vi "Dialog GraphSetting (Chart).vi"(11 "波形チャートref(in)":refnum<vi>) -> ()   [LabVIEW 2016]
uses:
  TypeDef/GraphSetting Appearance.ctl
  TypeDef/GraphSetting Plot.ctl
  SupportVIs/GraphSetting Scale.ctl
  TypeDef/GraphSetting DisplayFormatType.ctl
  TypeDef/GraphSetting All.ctl
  TypeDef/GraphSetting Command.ctl
  Library/Event/Write User Event (Array).vi
  <vilib>/Utility/xml.llb/Write to XML File(string).vi
  <vilib>/Utility/xml.llb/Read From XML File(string).vi
panel:
  in  "ファイル読込":bool
  in  "ファイル保存":bool
  in  "タブ制御器":enum32{"外観", "スケール", "プロット"}(tab)
  in  "外観":T1
  in  "Yスケール選択":u16(ring) items=["振幅"]
  in  "スケール(Y軸)":T2
  in  "スケール(X軸)":T2
  in  "Xスケール選択":u16(ring) items=["時間"]
  in  "プロット":T4 {"Yスケール" items=["振幅"]; "Xスケール" items=["時間"]; "プロット補間" max=5 step=1; "ポイントスタイル" max=16 step=1; "太さ" max=5 step=1; "ラインスタイル" max=4 step=1}
  in  "プロット選択":u16(ring) items=["正弦波", "プロット1"]
  in  "停止ボタン":bool
  # "欄外、パラメータ"
  # "スケールのスタイルとカラー"
  # "スケール係数"
  # "スケールのスタイルとカラー"
  # "スケールのスタイルとカラー"
  # "スケール係数"
  # "スケールのスタイルとカラー"
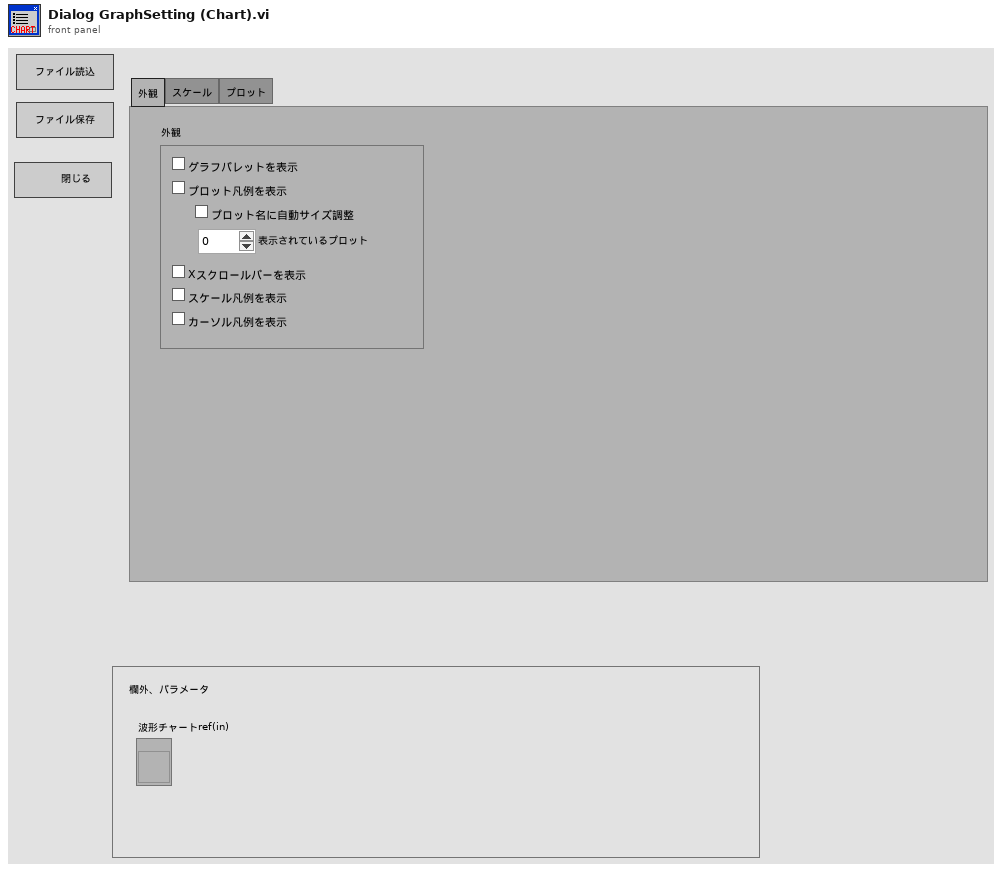
[diagram p1: front panel]
types:
  T1 = typedef "GraphSetting Appearance.ctl" = cluster{"グラフパレットを表示":bool, "プロット凡例を表示":bool, "プロット名に自動サイズ調整":bool, "表示されているプロット":u32, "Xスクロールバーを表示":bool, "スケール凡例を表示":bool, "カーソル凡例を表示":bool}
  T2 = typedef "GraphSetting Scale.ctl" = cluster{"名前":string, "スケールラベルを表示":bool, "スケールを表示":bool, "ログ":bool, "反転":bool, "自動スケール":bool, "最小":dbl, "最大":dbl, "オフセット":dbl, "乗数":dbl, "主目盛り":u32, "補助目盛り":u32, "マーカテキスト":u32, "主グリッド":u32, "補助グリッド":u32, "タイプ":T3, "小数点以下桁数":u8}
  T3 = typedef "GraphSetting DisplayFormatType.ctl" = enum8{"浮動小数点", "科学", "工学", "バイナリ", "８進数", "１６進数", "相対時間", "時間と日時", "SI"}
  T4 = typedef "GraphSetting Plot.ctl" = cluster{"名前":string, "表示":bool, "ラインスタイル":u8, "太さ":u8, "ポイントスタイル":u8, "プロット補間":u8, "ラインカラー":u32, "ポイント/塗りつぶし":u32, "Xスケール":u16, "Yスケール":u16}
  T5 = typedef "GraphSetting All.ctl" = cluster{"外観":T1, "スケールX[]":T2[], "スケールY[]":T2[], "プロット[]":T4[]}
  T6 = typedef "GraphSetting Command.ctl" = enum16{"Get(ref->ctl)", "Set(ctl->ref)"}
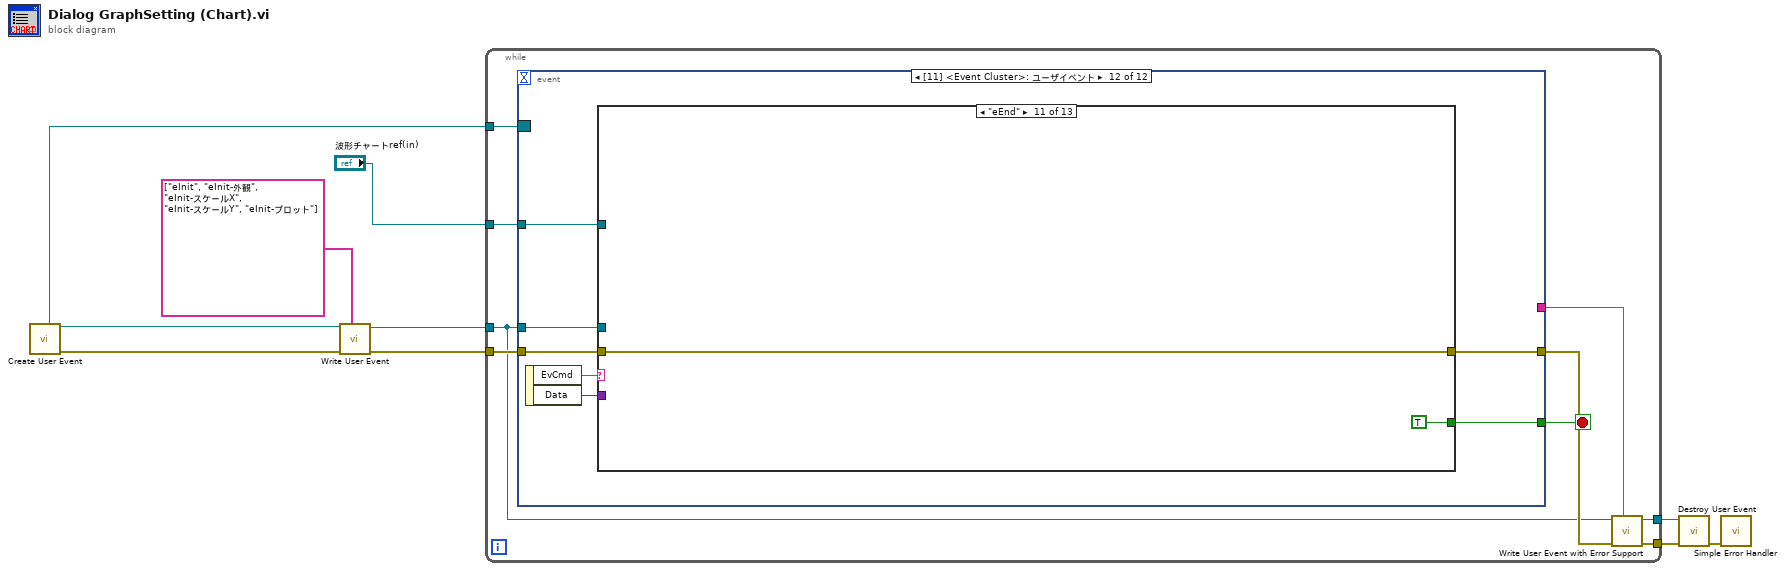
[diagram p0: block diagram]
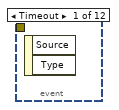
[diagram p2: hidden frame]
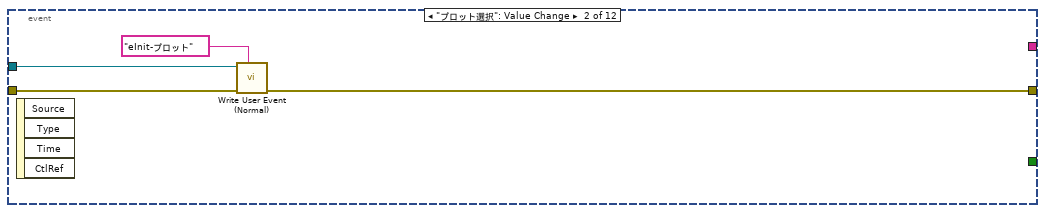
[diagram p3: hidden frame]
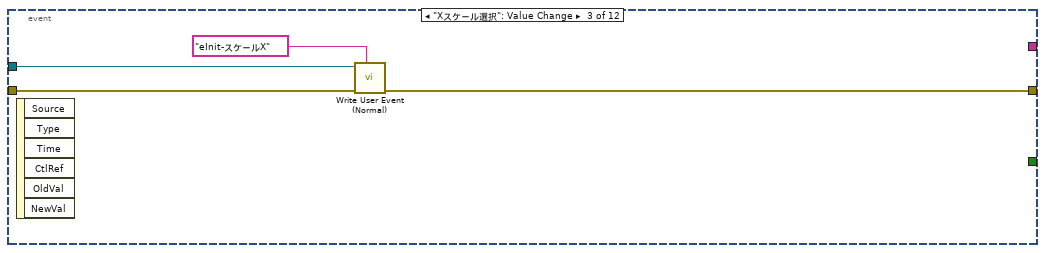
[diagram p4: hidden frame]
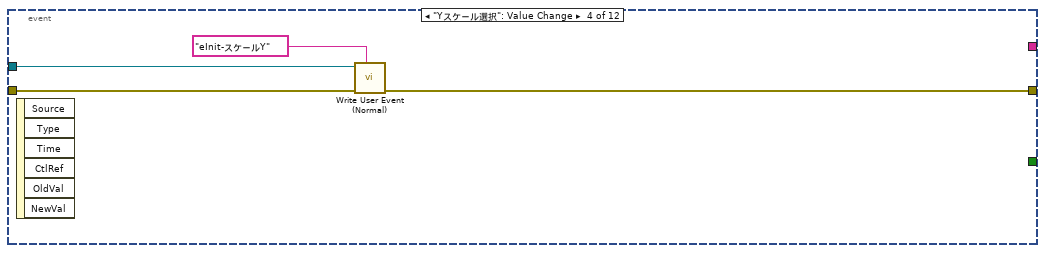
[diagram p5: hidden frame]
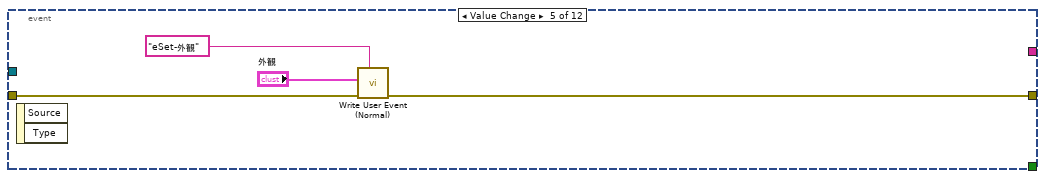
[diagram p6: hidden frame]
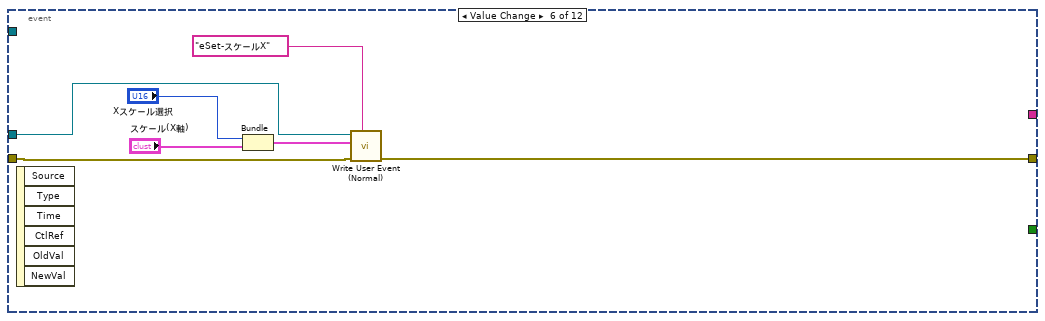
[diagram p7: hidden frame]
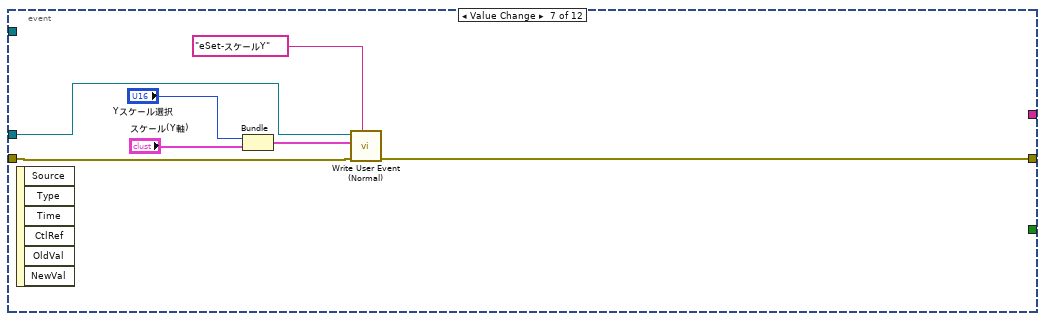
[diagram p8: hidden frame]
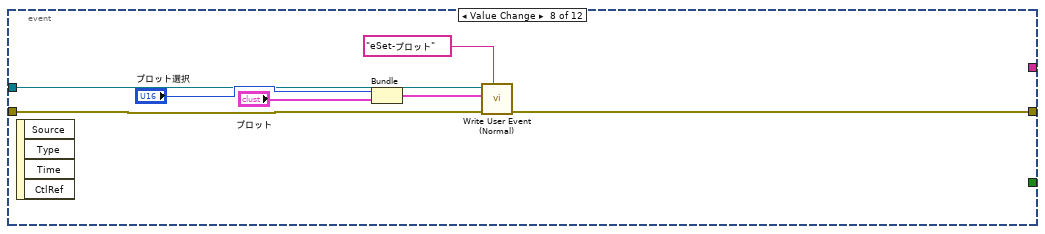
[diagram p9: hidden frame]
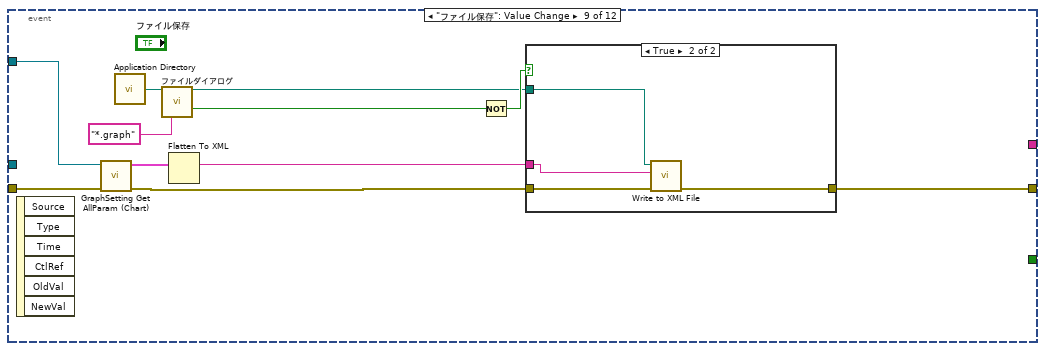
[diagram p10: hidden frame]
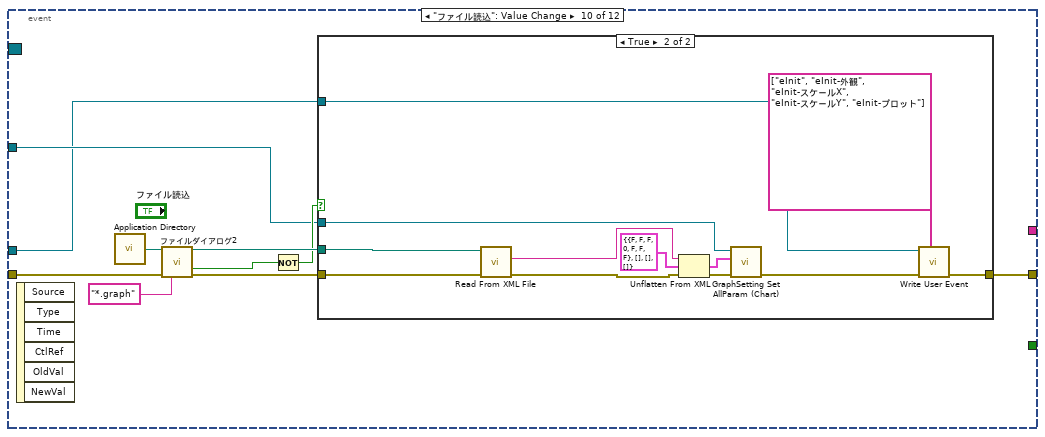
[diagram p12: hidden frame]
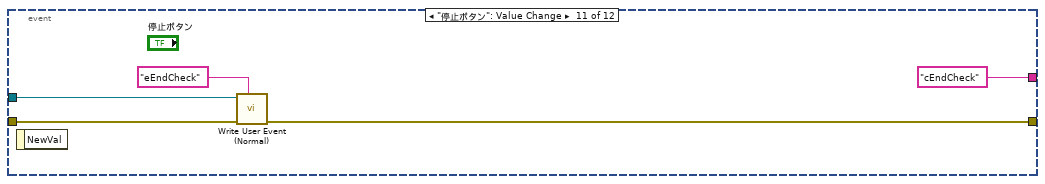
[diagram p14: hidden frame]
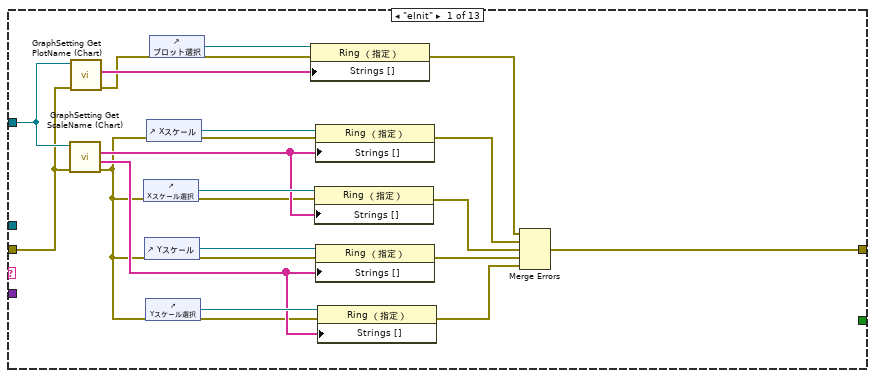
[diagram p15: hidden frame]
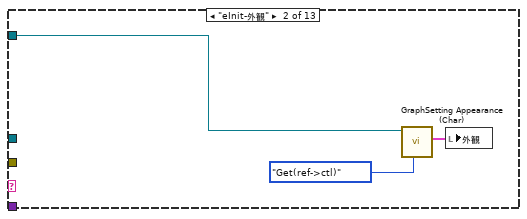
[diagram p16: hidden frame]
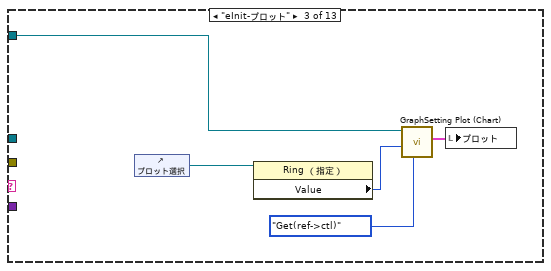
[diagram p17: hidden frame]
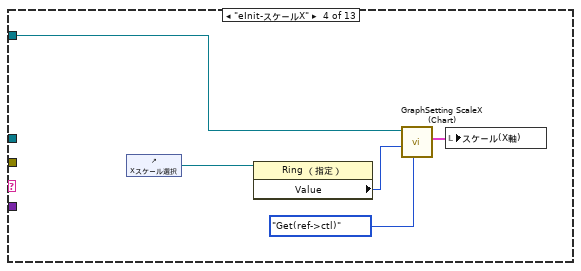
[diagram p18: hidden frame]
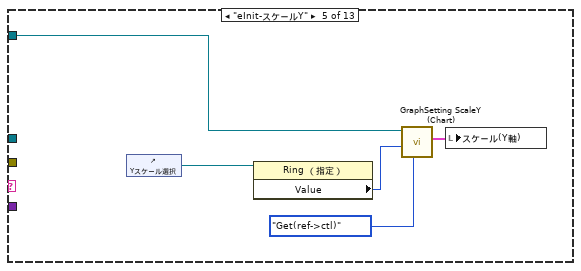
[diagram p19: hidden frame]
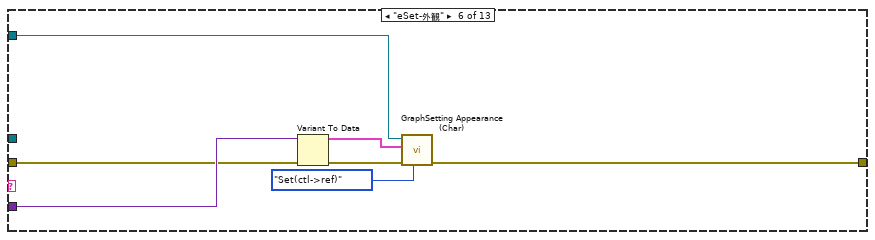
[diagram p20: hidden frame]
diagram:
  n1 = call "Create User Event.vi"() -> ("error out"=w8:errorcluster, "User Event"=w9:refnum<user-event>, "Event Registration Refnum"=w10:refnum<event-registration>)  [unwired: 9 in]
  n2 = call-poly "Write User Event.vi"("EvCmd[]"=string[] ["eInit", "eInit-外観", "eInit-スケールX", "eInit-スケールY", "eInit-プロット"], "エラー入力（エラーなし）"=w8, "ユーザイベント入力"=w9) -> ("エラー出力"=w4:errorcluster, "ユーザイベント出力"=w5:refnum<user-event>)  [unwired: 7 in]
  n3 = while {
    tunnel: w4 -> [w18]
    tunnel: w10 -> [w19]
    tunnel: [w15] -> w7
    tunnel: w5 -> [w11]
    tunnel: "波形チャートref(in)" -> [w17]
    tunnel: [w12] -> w2
    stop <- w13 stop-if-true
    n4 = event shown="[11] <Event Cluster>: ユーザイベント" {
      selector: w19 -> [_ _ _ _ _ _ _ _ _ _ _ _]
      dyn-events: _ -> [_ _ _ _ _ _ _ _ _ _ _ _]
      timeout: _ -> [_ _ _ _ _ _ _ _ _ _ _ _]
      tunnel: [_ _ _ _ _ _ _ _ _ _ _ w103] -> w13
      tunnel: [_ w21 w25 w28 w32 w37 w44 w51 w57 w74 w97 w104] -> w16
      tunnel: w18 -> [_ w22 w27 w30 w33 w36 w45 w52 w66 w80 w99 w105]
      tunnel: w11 -> [_ w23 w26 w29 _ w40 w46 w53 _ w73 w100 w102]
      tunnel: w17 -> [_ _ _ _ _ _ _ _ w67 w75 _ w101]
      tunnel: [_ _ _ _ _ _ _ _ _ _ "cEndCheck" _] -> w14
      event Timeout {
        n5 = event-data() -> ()  [unwired: 1 in, 2 out]
      }
      event "プロット選択": Value Change {
        n6 = event-data() -> ()  [unwired: 1 in, 4 out]
        n7 = call "Write User Event (Normal).vi"("EvCmd"="eInit-プロット", "エラー入力（エラーなし）"=w22, "ユーザイベント入力"=w23) -> ("エラー出力"=w21:errorcluster)  [unwired: 7 in, 1 out]
      }
      event "Xスケール選択": Value Change {
        n8 = event-data() -> ()  [unwired: 1 in, 6 out]
        n9 = call "Write User Event (Normal).vi"("EvCmd"="eInit-スケールX", "エラー入力（エラーなし）"=w27, "ユーザイベント入力"=w26) -> ("エラー出力"=w25:errorcluster)  [unwired: 7 in, 1 out]
      }
      event "Yスケール選択": Value Change {
        n10 = event-data() -> ()  [unwired: 1 in, 6 out]
        n11 = call "Write User Event (Normal).vi"("EvCmd"="eInit-スケールY", "エラー入力（エラーなし）"=w30, "ユーザイベント入力"=w29) -> ("エラー出力"=w28:errorcluster)  [unwired: 7 in, 1 out]
      }
      event Value Change {
        n12 = event-data() -> ()  [unwired: 1 in, 2 out]
        n13 = call "Write User Event (Normal).vi"("EvCmd"="eSet-外観", "エラー入力（エラーなし）"=w33, "データ"="外観") -> ("エラー出力"=w32:errorcluster)  [unwired: 7 in, 1 out]
      }
      event Value Change {
        n14 = event-data() -> ()  [unwired: 1 in, 6 out]
        n15 = Bundle("Xスケール選択"="Xスケール選択", "スケール(X軸)"="スケール(X軸)") -> (w41:cluster{"Xスケール選択":u16, "スケール(X軸)":T2})  [unwired: 1 in]
        n16 = call "Write User Event (Normal).vi"("EvCmd"="eSet-スケールX", "エラー入力（エラーなし）"=w36, "データ"=w41, "ユーザイベント入力"=w40) -> ("エラー出力"=w37:errorcluster)  [unwired: 6 in, 1 out]
      }
      event Value Change {
        n17 = event-data() -> ()  [unwired: 1 in, 6 out]
        n18 = Bundle("Yスケール選択"="Yスケール選択", "スケール(Y軸)"="スケール(Y軸)") -> (w47:cluster{"Yスケール選択":u16, "スケール(Y軸)":T2})  [unwired: 1 in]
        n19 = call "Write User Event (Normal).vi"("EvCmd"="eSet-スケールY", "エラー入力（エラーなし）"=w45, "データ"=w47, "ユーザイベント入力"=w46) -> ("エラー出力"=w44:errorcluster)  [unwired: 6 in, 1 out]
      }
      event Value Change {
        n20 = event-data() -> ()  [unwired: 1 in, 4 out]
        n21 = Bundle("プロット選択"="プロット選択", "プロット"="プロット") -> (w54:cluster{"プロット選択":u16, "プロット":T4})  [unwired: 1 in]
        n22 = call "Write User Event (Normal).vi"("EvCmd"="eSet-プロット", "エラー入力（エラーなし）"=w52, "データ"=w54, "ユーザイベント入力"=w53) -> ("エラー出力"=w51:errorcluster)  [unwired: 6 in, 1 out]
      }
      event "ファイル保存": Value Change {
        n23 = event-data() -> ()  [unwired: 1 in, 6 out]
        n24 = call "GraphSetting Get AllParam (Chart).vi"("エラー入力（エラーなし）"=w66, "WaveformChart入力"=w67) -> ("エラー出力"=w59:errorcluster, "クラスタ"=w58:cluster{"外観(out)":T1, T2[], T2[], T4[]})  [unwired: 8 in]
        n25 = call <vilib>:"Application Directory.vi"() -> ("Application Directory"=w64:path)
        n26 = call "ファイルダイアログ"("start path"=w64, "pattern (all files)"="*.graph") -> ("selected path"=w60:path, "cancelled"=w61:bool)  [unwired: 10 in, 2 out]
        n27 = Flatten To XML(anything=w58) -> (xml string=w62:string)
        n28 = Not(x=w61) -> (.not. x?=w63:bool)
        n29 = case shown="TRUE" w63 {
          tunnel: w60 -> [_ w72]
          tunnel: w62 -> [_ w71]
          tunnel: w59 -> [w68 w69]
          tunnel: [w68 w70] -> w57
          frame False {
          }
          frame True {
            n30 = call-poly <vilib>:"Write to XML File.vi"("error in (no error)"=w69, "XML Input"=w71, "XML File Path"=w72) -> ("error out"=w70:errorcluster)  [unwired: 6 in, 2 out]
          }
        }
      }
      event "ファイル読込": Value Change {
        n31 = event-data() -> ()  [unwired: 1 in, 6 out]
        n32 = call <vilib>:"Application Directory.vi"() -> ("Application Directory"=w82:path)
        n33 = call "ファイルダイアログ2"("start path"=w82, "error in"=w80, "pattern (all files)"="*.graph") -> ("selected path"=w79:path, "cancelled"=w78:bool, "error out"=w76:errorcluster)  [unwired: 9 in, 1 out]
        n34 = Not(x=w78) -> (.not. x?=w77:bool)
        n35 = case shown="TRUE" w77 {
          tunnel: w79 -> [_ w93]
          tunnel: w76 -> [w83 w91]
          tunnel: w75 -> [_ w88]
          tunnel: [w83 w85] -> w74
          tunnel: w73 -> [_ w87]
          frame False {
          }
          frame True {
            n36 = call-poly <vilib>:"Read From XML File.vi"("error in (no error)"=w91, "XML File Path"=w93) -> ("error out"=w92:errorcluster, "XML Elements"=w94:string)  [unwired: 7 in, 1 out]
            n37 = Unflatten From XML(xml string=w94, type=T5 {"外観"={"グラフパレットを表示"=FALSE, "プロット凡例を表示"=FALSE, "プロット名に自動サイズ調整"=FALSE, "表示されているプロット"=0, "Xスクロールバーを表示"=FALSE, "スケール凡例を表示"=FALSE, "カーソル凡例を表示"=FALSE}, "スケールX[]"=[], "スケールY[]"=[], "プロット[]"=[]} ("出力クラスタ"), error in (no error)=w92) -> (value=w90:T5, error out=w89:errorcluster)
            n38 = call "GraphSetting Set AllParam (Chart).vi"("error in (no error)"=w89, "Chartグラフパラメータ"=w90, "波形チャートref(in)"=w88) -> ("error out"=w86:errorcluster)  [unwired: 8 in]
            n39 = call-poly "Write User Event.vi"("EvCmd[]"=string[] ["eInit", "eInit-外観", "eInit-スケールX", "eInit-スケールY", "eInit-プロット"], "エラー入力（エラーなし）"=w86, "ユーザイベント入力"=w87) -> ("エラー出力"=w85:errorcluster)  [unwired: 7 in, 1 out]
          }
        }
      }
      event "停止ボタン": Value Change {
        n40 = event-data() -> ()  [unwired: 1 in, 1 out]
        n41 = call "Write User Event (Normal).vi"("EvCmd"="eEndCheck", "エラー入力（エラーなし）"=w99, "ユーザイベント入力"=w100) -> ("エラー出力"=w97:errorcluster)  [unwired: 7 in, 1 out]
      }
      event User Event {
        n42 = event-data() -> ("EvCmd"=w107:string, "Data"=w106:variant)  [unwired: 1 in]
        n43 = case shown="\"eEnd\"" w107 {
          selector: w107 -> [_ _ _ _ _ _ _ _ _ _ _ _ w191]
          tunnel: w106 -> [_ _ _ _ _ w148 w156 w167 w177 _ _ w190 _]
          tunnel: w105 -> [w117 _ _ _ _ w146 w158 w166 w176 w181 w185 w188 _]
          tunnel: [w108 _ _ _ _ w144 w151 w160 w170 w180 w185 _ _] -> w104
          tunnel: [_ _ _ _ _ _ _ _ _ _ TRUE TRUE _] -> w103
          tunnel: w102 -> [_ _ _ _ _ _ _ _ _ w183 _ _ _]
          tunnel: w101 -> [w120 w128 w133 w138 w143 w149 w152 w164 w174 _ _ _ _]
          frame "eInit" {
            n44 = call "GraphSetting Get ScaleName (Chart).vi"("error in (no error)"=w117, "波形チャートref(in)"=w120) -> ("error out"=w114:errorcluster, "Y軸名称[]"=w116:string[], "X軸名称[]"=w123:string[])  [unwired: 7 in]
            n45 = call "GraphSetting Get PlotName (Chart).vi"("error in (no error)"=w117, "波形チャートref(in)"=w120) -> ("error out"=w115:errorcluster, "プロット名称[]"=w118:string[])  [unwired: 8 in]
            n46 = control-ref of="Xスケール選択"() -> (w124:refnum<vi>)
            n47 = control-ref of="Yスケール"() -> (w121:refnum<vi>)
            n48 = control-ref of="Yスケール選択"() -> (w122:refnum<vi>)
            n49 = control-ref of="Xスケール"() -> (w125:refnum<vi>)
            n50 = control-ref of="プロット選択"() -> (w119:refnum<vi>)
            n51 = property class="Ring （指定）"(reference=w119, error in=w115, "Strings []"=w118) -> (error out=w113:errorcluster)  [unwired: 1 out]
            n52 = property class="Ring （指定）"(reference=w124, error in=w114, "Strings []"=w123) -> (error out=w111:errorcluster)  [unwired: 1 out]
            n53 = property class="Ring （指定）"(reference=w125, error in=w114, "Strings []"=w123) -> (error out=w112:errorcluster)  [unwired: 1 out]
            n54 = property class="Ring （指定）"(reference=w121, error in=w114, "Strings []"=w116) -> (error out=w110:errorcluster)  [unwired: 1 out]
            n55 = property class="Ring （指定）"(reference=w122, error in=w114, "Strings []"=w116) -> (error out=w109:errorcluster)  [unwired: 1 out]
            n56 = Merge Errors(w113, w112, w111, w110, w109) -> (w108:errorcluster)
          }
          frame "eInit-外観" {
            n57 = call "GraphSetting Appearance (Char).vi"("コマンド"=GraphSetting_Command."Get(ref->ctl)", "WaveformChart入力"=w128) -> ("外観(out)"=w127:T1)  [unwired: 8 in, 1 out]
            n58 = local write "外観"(w127) -> ()
          }
          frame "eInit-プロット" {
            n59 = control-ref of="プロット選択"() -> (w132:refnum<vi>)
            n60 = property class="Ring （指定）"(reference=w132) -> ("Value"=w131:u16)  [unwired: 1 in, 2 out]
            n61 = call "GraphSetting Plot (Chart).vi"("コマンド"=GraphSetting_Command."Get(ref->ctl)", "アクティブプロット"=w131, "波形チャートref(in)"=w133) -> ("プロット(out)"=w129:T4)  [unwired: 7 in, 1 out]
            n62 = local write "プロット"(w129) -> ()
          }
          frame "eInit-スケールX" {
            n63 = control-ref of="Xスケール選択"() -> (w137:refnum<vi>)
            n64 = property class="Ring （指定）"(reference=w137) -> ("Value"=w136:u16)  [unwired: 1 in, 2 out]
            n65 = call "GraphSetting ScaleX (Chart).vi"("コマンド"=GraphSetting_Command."Get(ref->ctl)", "アクティブスケール(X)"=w136, "波形チャートref(in)"=w138) -> ("スケール(out)"=w134:T2)  [unwired: 7 in, 1 out]
            n66 = local write "スケール(X軸)"(w134) -> ()
          }
          frame "eInit-スケールY" {
            n67 = control-ref of="Yスケール選択"() -> (w142:refnum<vi>)
            n68 = property class="Ring （指定）"(reference=w142) -> ("Value"=w141:u16)  [unwired: 1 in, 2 out]
            n69 = call "GraphSetting ScaleY (Chart).vi"("コマンド"=GraphSetting_Command."Get(ref->ctl)", "アクティブスケールY"=w141, "波形チャートref(in)"=w143) -> ("スケール(out)"=w139:T2)  [unwired: 7 in, 1 out]
            n70 = local write "スケール(Y軸)"(w139) -> ()
          }
          frame "eSet-外観" {
            n71 = Variant To Data(error in=w146, Variant=w148) -> (data=w147:T1, error out=w145:errorcluster)  [unwired: 1 in]
            n72 = call "GraphSetting Appearance (Char).vi"("コマンド"=GraphSetting_Command."Set(ctl->ref)", "error in (no error)"=w145, "外観(in)"=w147, "WaveformChart入力"=w149) -> ("error out"=w144:errorcluster)  [unwired: 6 in, 1 out]
          }
          frame "eSet-スケールX" {
            n73 = Variant To Data(type=cluster{"Xスケール選択":u16, "スケール(X軸)":T2} {"Xスケール選択"=0, "スケール(X軸)"={"名前"="", "スケールラベルを表示"=FALSE, "スケールを表示"=FALSE, "ログ"=FALSE, "反転"=FALSE, "自動スケール"=FALSE, "最小"=0.0, "最大"=0.0, "オフセット"=0.0, "乗数"=0.0, "主目盛り"=0, "補助目盛り"=0, "マーカテキスト"=0, "主グリッド"=0, "補助グリッド"=0, "タイプ"=enum."浮動小数点", "小数点以下桁数"=0}} ("出力クラスタ"), Variant=w156) -> (data=w155:cluster{"Xスケール選択":u16, "スケール(X軸)":T2})  [unwired: 1 in, 1 out]
            n74 = Unbundle(w155) -> ("Xスケール選択"=w153:u16, "スケール(X軸)"=w154:T2)
            n75 = call "GraphSetting ScaleX (Chart).vi"("コマンド"=GraphSetting_Command."Set(ctl->ref)", "error in (no error)"=w158, "アクティブスケール(X)"=w153, "スケール(in)"=w154, "波形チャートref(in)"=w152) -> ("error out"=w151:errorcluster)  [unwired: 5 in, 1 out]
          }
          frame "eSet-スケールY" {
            n76 = Variant To Data(error in=w166, type=cluster{"Xスケール選択":u16, "スケール(X軸)":T2} {"Xスケール選択"=0, "スケール(X軸)"={"名前"="", "スケールラベルを表示"=FALSE, "スケールを表示"=FALSE, "ログ"=FALSE, "反転"=FALSE, "自動スケール"=FALSE, "最小"=0.0, "最大"=0.0, "オフセット"=0.0, "乗数"=0.0, "主目盛り"=0, "補助目盛り"=0, "マーカテキスト"=0, "主グリッド"=0, "補助グリッド"=0, "タイプ"=enum."浮動小数点", "小数点以下桁数"=0}} ("出力クラスタ"), Variant=w167) -> (data=w165:cluster{"Xスケール選択":u16, "スケール(X軸)":T2}, error out=w161:errorcluster)
            n77 = Unbundle(w165) -> ("Xスケール選択"=w162:u16, "スケール(X軸)"=w163:T2)
            n78 = call "GraphSetting ScaleY (Chart).vi"("コマンド"=GraphSetting_Command."Set(ctl->ref)", "error in (no error)"=w161, "アクティブスケールY"=w162, "スケール(in)"=w163, "波形チャートref(in)"=w164) -> ("error out"=w160:errorcluster)  [unwired: 5 in, 1 out]
          }
          frame "eSet-プロット" {
            n79 = Variant To Data(error in=w176, type=cluster{"プロット選択":u16, "プロット":T4} {"プロット選択"=0, "プロット"={"名前"="", "表示"=FALSE, "ラインスタイル"=0, "太さ"=0, "ポイントスタイル"=0, "プロット補間"=0, "ラインカラー"=0, "ポイント/塗りつぶし"=0, "Xスケール"=0, "Yスケール"=0}} ("出力クラスタ"), Variant=w177) -> (data=w175:cluster{"プロット選択":u16, "プロット":T4}, error out=w173:errorcluster)
            n80 = Unbundle(w175) -> ("プロット選択"=w172:u16, "プロット"=w171:T4)
            n81 = call "GraphSetting Plot (Chart).vi"("コマンド"=GraphSetting_Command."Set(ctl->ref)", "error in (no error)"=w173, "アクティブプロット"=w172, "プロット(in)"=w171, "波形チャートref(in)"=w174) -> ("error out"=w170:errorcluster)  [unwired: 5 in, 1 out]
          }
          frame "eEndCheck" {
            n82 = call "Write User Event (Normal).vi"("EvCmd"="eEnd", "エラー入力（エラーなし）"=w181, "ユーザイベント入力"=w183) -> ("エラー出力"=w180:errorcluster)  [unwired: 7 in, 1 out]
          }
          frame "eEnd" {
          }
          frame "eError" {
            n83 = Variant To Data(error in=w188, type=errorcluster {"status"=FALSE, "code"=0, "source"=""} ("エラー定数"), Variant=w190) -> (data=w187:errorcluster)  [unwired: 1 out]
            n84 = call <vilib>:"Simple Error Handler.vi"("error in (no error)"=w187) -> ()  [unwired: 4 in, 5 out]
          }
          frame Default {
            n85 = call "DialogProgramError.vi"("エラー内容"="ユーザイベント例外" ("エラー詳細"), "エラー詳細"=w191) -> ()  [unwired: 9 in, 1 out]
          }
        }
      }
    }
    n86 = call "Write User Event with Error Support.vi"("EvCmd"=w14, "エラー入力（エラーなし）"=w16, "ユーザイベント入力"=w11) -> ("エラー出力"=w15:errorcluster, "ユーザイベント出力"=w12:refnum<user-event>)  [unwired: 7 in]
  }
  n87 = call "Destroy User Event.vi"("error in (no error)"=w7, "User Event"=w2) -> ("error out"=w6:errorcluster)  [unwired: 9 in]
  n88 = call <vilib>:"Simple Error Handler.vi"("error in (no error)"=w6) -> ()  [unwired: 4 in, 5 out]
